vi "Update Object.vi"(11 "Scene in":refnum<class "Scene.lvclass">) -> (3 "Scene out":refnum<class "Scene.lvclass">)   [LabVIEW 2020, in "Scene.lvclass"]
uses:
  Scene.lvclass
  Scene.lvclass/Scene.ctl
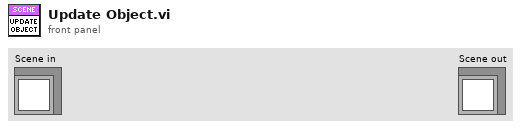
[diagram p1: front panel]
types:
  T1 = typedef "3D.lvlib/Transform.ctl" = cluster{"Position":T2, "Rotation":T2, "Scale":T2}
  T2 = typedef "3D.lvlib/Vector 3D.ctl" = cluster{"x":sgl, "y":sgl, "z":sgl}
  T3 = typedef "3D.lvlib/Object.ctl" = cluster{"Triangles":T4[], "Transform":T1, "Name":string, "Alpha Blending Enabled":bool, "Alpha":dbl, "Turntable Enabled":bool, "Material":T7}
  T4 = typedef "3D.lvlib/Triangle.ctl" = cluster{"Vertex 1":T5, "Vertex 2":T5, "Vertex 3":T5, "Alpha":dbl, "Alpha Blending Enabled":bool, "Colour":u32, "Material":T7}
  T5 = typedef "3D.lvlib/Vertex.ctl" = cluster{"Position":T2, "UV":T6, "Colour":u32}
  T6 = typedef "Raster.lvlib/UV.ctl" = cluster{"u":sgl, "v":sgl}
  T7 = typedef "3D.lvlib/Material.ctl" = cluster{"Diffuse Colour":u32, "Texture":T8}
  T8 = typedef "Raster.lvlib/Texture.ctl" = cluster{"Pixels":refnum<data-value>, "Size":T9}
  T9 = typedef "Raster.lvlib/Rectangle Dimensions.ctl" = cluster{"Width":u32, "Height":u32}
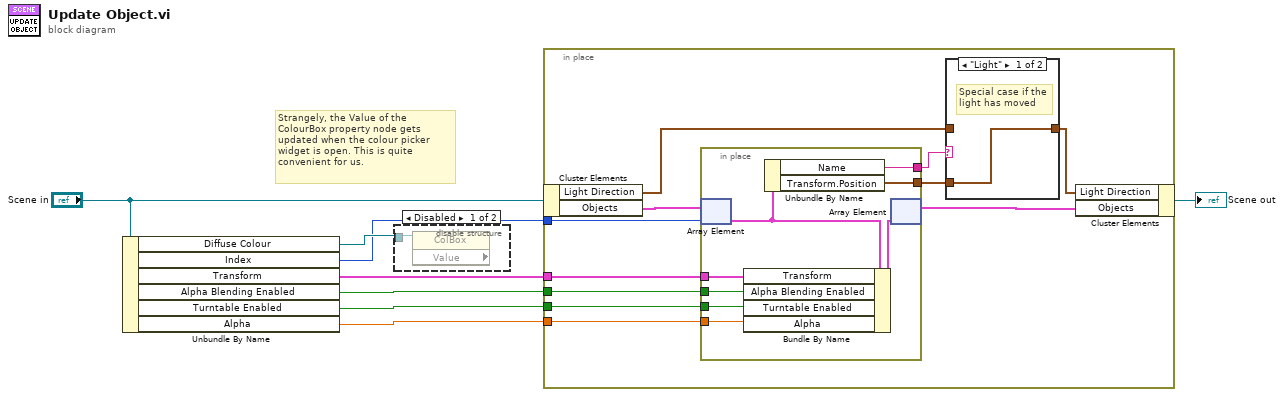
[diagram p0: block diagram]
diagram:
  # "Strangely, the Value of the ColourBox property node gets updated when the colour picker widget is open. This is quite convenient for us."
  n1 = Unbundle By Name("Scene in") -> ("Diffuse Colour"=w6:refnum<vi>, "Index"=w5:i32, "Transform"=w3:T1, "Alpha Blending Enabled"=w4:bool, "Turntable Enabled"=w2:bool, "Alpha"=w1:dbl)
  n2 = disable-structure shown="Disabled" {
    disable-tunnel: w6 -> [w9 _]
    frame Disabled {
      n3 = property class="ColBox" props=["Value"](reference=w9) -> ()  [unwired: 1 in, 3 out]
    }
    frame Enabled {
    }
  }
  n4 = in-place {
    in-place-border: w5 -> [w19]
    in-place-border: w3 -> [w17]
    in-place-border: w4 -> [w12]
    in-place-border: w2 -> [w11]
    in-place-border: w1 -> [w10]
    n5 = in-place-cluster #1("Scene in") -> ("Light Direction"=w14:T2, "Objects"=w20:T3[])
    n6 = in-place {
      in-place-border: w17 -> [w29]
      in-place-border: [w27] -> w16
      in-place-border: [w26] -> w13
      in-place-border: w12 -> [w25]
      in-place-border: w11 -> [w24]
      in-place-border: w10 -> [w23]
      n7 = in-place-array #2(w20, w19) -> (w28:T3)
      n8 = Bundle By Name(cluster=w28, "Transform"=w29, "Alpha Blending Enabled"=w25, "Turntable Enabled"=w24, "Alpha"=w23) -> (w30:T3)
      n9 = Unbundle By Name(w28) -> ("Name"=w27:string, "Transform.Position"=w26:T2)
      n10 = in-place-array #2(w30) -> (w18:T3[])  [unwired: 1 out]
    }
    n11 = case shown="\"Light\"" w16 {
      tunnel: [w21 w22] -> w15
      tunnel: w14 -> [_ w22]
      tunnel: w13 -> [w21 _]
      frame "Light" {
        # "Special case if the light has moved"
      }
      frame Default {
      }
    }
    n12 = in-place-cluster #1("Light Direction"=w15, "Objects"=w18) -> (→"Scene out":refnum<class "Scene.lvclass">)
  }
